vi "Begin.vi"(5 "_oscillator_freq":u32, 7 "I2C Chanel(1)":i32=1, 8 "error in (no error)":errorcluster, 9 "_freq":sgl, 10 "LINX Resource":T1, 11 "Motorshield in":refnum<class "Motorshield.lvclass">) -> (0 "error out":errorcluster, 2 "OK":bool=TRUE, 3 "Motorshield out":refnum<class "Motorshield.lvclass">)   [LabVIEW 2022 SP3, in "Motorshield.lvlib" / "Motorshield.lvclass"]
uses:
  Motorshield.lvclass
  <vilib>/MakerHub/LINX/Private/Type Defs/LINX Ref.ctl
  <vilib>/MakerHub/LINX/Private/Type Defs/Platform.ctl
  <vilib>/MakerHub/LINX/Private/Type Defs/Interface.ctl
  <vilib>/MakerHub/LINX/Private/Device/Type Defs/LINX Device Config.ctl
  <vilib>/MakerHub/LINX/Private/Device/Type Defs/TCP Config.ctl
  <vilib>/MakerHub/LINX/Private/Device/Type Defs/Channels.ctl
  Motorshield.lvclass/Motorshield.ctl
  pca985/PCA/PCA.lvclass
  <vilib>/MakerHub/LINX/LMH-LINX.lvlib
  <vilib>/MakerHub/LINX/Private/Device/Device.lvlib
panel:
  out "Boolean":bool
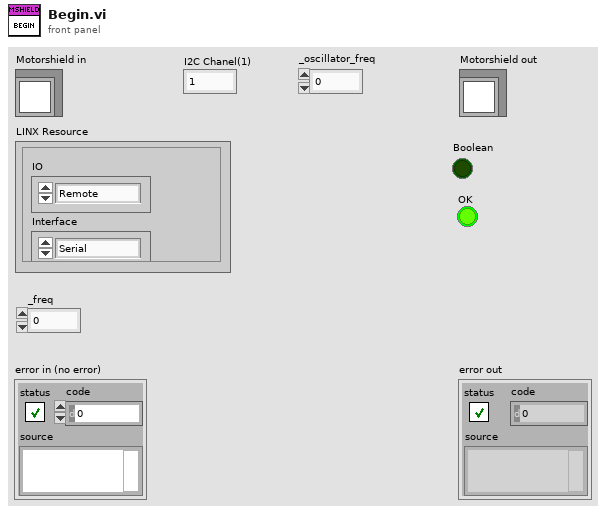
[diagram p1: front panel]
types:
  T1 = typedef "LMH-LINX.lvlib/LINX Ref.ctl" = cluster{"IO":T2, "Interface":T3, "LINX Device Config":T4}
  T2 = typedef "LMH-LINX.lvlib/Platform.ctl" = enum16{"Remote", "Local"}
  T3 = typedef "LMH-LINX.lvlib/Interface.ctl" = enum16{"Serial", "TCP"}
  T4 = typedef "LMH-LINX.lvlib/Device.lvlib/LINX Device Config.ctl" = cluster{"Interface":T3, "COM Port":refnum<visa-resource-name>, "TCP Configuration":T5, "Device Family":u8, "Device ID":u8, "Device Name":string, "TCP Ref":refnum<k5>, "Channels":T6}
  T5 = typedef "LMH-LINX.lvlib/Device.lvlib/TCP Config.ctl" = cluster{"IP Address":string, "Port":u16}
  T6 = typedef "LMH-LINX.lvlib/Channels.ctl" = cluster{"DI":u8[], "DO":u8[], "AI":u8[], "AO":u8[], "PWM":u8[], "QE":u8[], "UART":u8[], "I2C 2":u8[], "SPI":u8[], "CAN":u8[], "Servo":u8[], "AI Ref (V)":dbl, "AI Resolution (Bits)":u8, "AO Ref (V)":dbl, "AO Resolution (Bits)":u8}
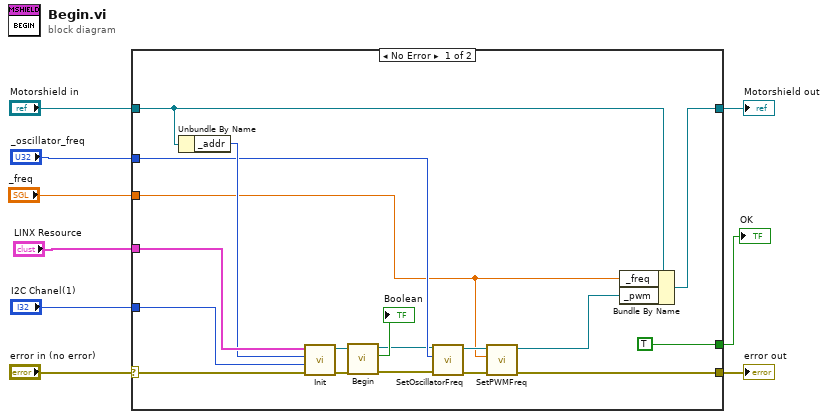
[diagram p0: block diagram]
diagram:
  n1 = case shown="No Error" "error in (no error)" {
    selector: "error in (no error)" -> [w27 w29]
    tunnel: [w10 w29] -> w8
    tunnel: [w22 w28] -> w6
    tunnel: "Motorshield in" -> [w24 w28]
    tunnel: "LINX Resource" -> [w26 _]
    tunnel: "I2C Chanel(1)" -> [w25 _]
    tunnel: "_freq" -> [w12 _]
    tunnel: [TRUE _] -> w2
    tunnel: "_oscillator_freq" -> [w17 _]
    frame No Error {
      n2 = Unbundle By Name(w24) -> ("_addr"=w23:u8)
      n3 = call "Init.vi"("error in (no error)"=w27, "I2C Chanel(1)"=w25, "I2C Slave Address (61)"=w23, "LINX Resource"=w26) -> ("error out"=w20:errorcluster, "PCA out"=w19:refnum<class "PCA.lvclass">)  [unwired: 6 in]
      n4 = call "Begin.vi"("error in (no error)"=w20, "PCA in"=w19) -> ("error out"=w15:errorcluster, "Boolean"=→"Boolean":bool, "PCA out"=w16:refnum<class "PCA.lvclass">)  [unwired: 7 in]
      n5 = call "SetOscillatorFreq.vi"("error in (no error)"=w15, "_oscillator_freq"=w17, "PCA in"=w16) -> ("error out"=w13:errorcluster, "PCA out"=w14:refnum<class "PCA.lvclass">)  [unwired: 7 in]
      n6 = call "SetPWMFreq.vi"("error in (no error)"=w13, "Freq"=w12, "PCA in"=w14) -> ("error out"=w10:errorcluster, "PCA out"=w11:refnum<class "PCA.lvclass">)  [unwired: 7 in]
      n7 = Bundle By Name(cluster=w24, "_freq"=w12, "_pwm"=w11) -> (w22:refnum<class "Motorshield.lvclass">)
    }
    frame Error {
    }
  }
  "error out" <- w8
  "Motorshield out" <- w6
  "OK" <- w2
